vi "Configure Soft Iron Compensation.vi"(8 "error in (no error)":errorcluster, 10 "Enable Soft Iron Compensation":bool, 11 "VISA resource name":refnum<visa-resource-name>) -> (0 "error out":errorcluster, 3 "VISA resource out":refnum<visa-resource-name>)   [LabVIEW 2011, in "Ocean Server OS4000.lvlib"]
doc: "Enable or Disable Soft Iron Compensation."
uses:
  Ocean Server OS4000.lvlib
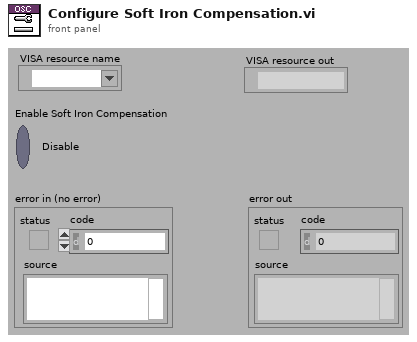
[diagram p1: front panel]
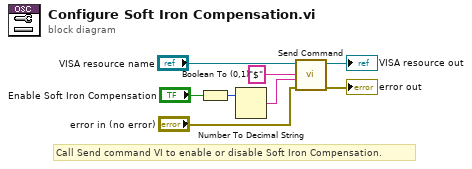
[diagram p0: block diagram]
diagram:
  # "Call Send command VI to enable or disable Soft Iron Compensation."
  n1 = Boolean To (0,1)(Boolean="Enable Soft Iron Compensation") -> (0, 1=w1:i16)
  n2 = Number To Decimal String(number=w1) -> (decimal integer string=w6:string)  [unwired: 1 in]
  n3 = call "Send Command.vi"("error in (no error)"="error in (no error)", "Value"=w6, "Message"="$", "VISA resource name"="VISA resource name") -> ("error out"=→"error out":errorcluster, "VISA resource out"=→"VISA resource out":refnum<visa-resource-name>)  [unwired: 6 in]
